vi "Configure Integration.vi"(7 "Independent Integration (F: Disable)":bool, 8 "error in (no error)":errorcluster, 9 "Auto Calibration (F: Disable)":bool, 10 "Integration Mode (0: Normal)":i32(ring) items=["Normal", "Continuous", "Real-time Normal", "Real-time Continuous"], 11 "VISA resource name":refnum<visa-resource-name>) -> (0 "error out":errorcluster, 3 "VISA resource name out":refnum<visa-resource-name>)   [LabVIEW 2021, in "Yokogawa WT1800 Series.lvlib"]
doc: "Configures the integrated power features."
uses:
  <instrlib>/Yokogawa WT1800 Series/Yokogawa WT1800 Series.lvlib
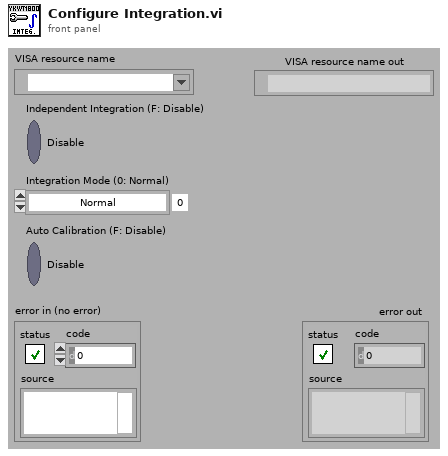
[diagram p1: front panel]
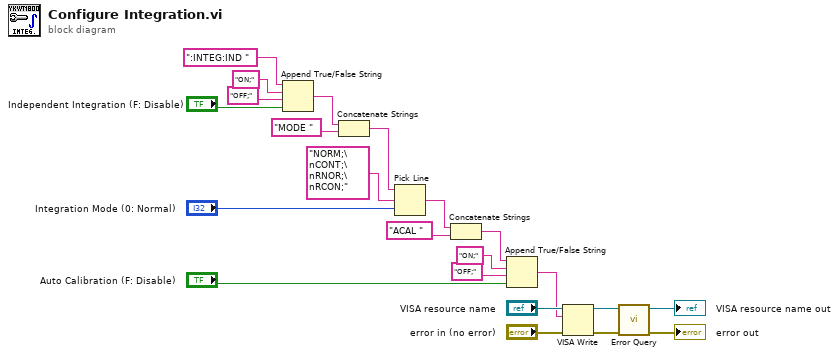
[diagram p0: block diagram]
diagram:
  n1 = Append True/False String ("True/False 文字列を追加")(1:"Independent Integration (F: Disable)", 2:"OFF;", 3:"ON;", 4:":INTEG:IND ") -> (0:w9:string)
  n2 = Concatenate Strings(w9, "MODE ") -> (w8:string)
  n3 = Pick Line ("ライン選択")(string ("")=w8, multi-line string="NORM;\nCONT;\nRNOR;\nRCON;" ("複数行文字列"), line index="Integration Mode (0: Normal)") -> (output string=w6:string)
  n4 = Concatenate Strings(w6, "ACAL ") -> (w5:string)
  n5 = Append True/False String ("True/False 文字列を追加")(1:"Auto Calibration (F: Disable)", 2:"OFF;", 3:"ON;", 4:w5) -> (0:w2:string)
  n6 = VISA Write ("VISA書き込み")(VISA resource name="VISA resource name", write buffer=w2, error in (no error)="error in (no error)") -> (VISA resource name out=w22:refnum<visa-resource-name>, error out=w21:errorcluster)  [unwired: 1 out]
  n7 = call <instrlib>:"Error Query.vi"("error in (no error)"=w21, "VISA resource name"=w22) -> ("error out"=→"error out":errorcluster, "VISA resource name out"=→"VISA resource name out":refnum<visa-resource-name>)  [unwired: 6 in, 2 out]
